vi "Init Splitter.vi"(4 "Maximal size":i16[](array[numeric]), 5 "Label":string, 6 "Minimal size":i16[](array[numeric]), 7 "Vertical? [F, hor.]":bool, 8 "error in (no error)":errorcluster, 9 "Relative size":dbl[](array[numeric]), 10 "Items":refnum<class "IObject.lvclass">[](array[class])) -> (0 "error out":errorcluster, 3 "Splitter out":refnum<class "Splitter.lvclass">)   [LabVIEW 2021, in "Splitter.lvclass"]
doc: "Copyright 2018, Wiebe Walstra, wiebe@carya.nl."
uses:
  Splitter.lvclass
  C:/Projects/Dynamic-Scaling/Dynamic Scaling/IContainer/Divider/Divider.lvclass
  IObject.lvclass
  Divider.lvclass
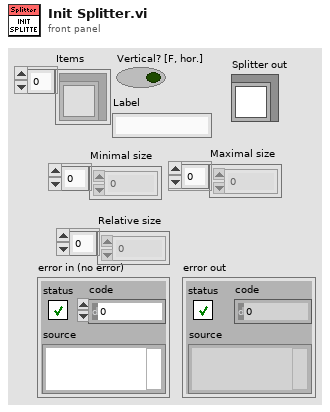
[diagram p1: front panel]
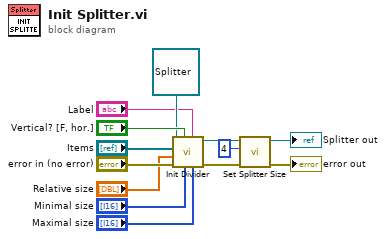
[diagram p0: block diagram]
diagram:
  n1 = call "Init Divider.vi"("Maximal size"="Maximal size", "Label"="Label", "Minimal size"="Minimal size", "Vertical? [F, hor.]"="Vertical? [F, hor.]", "error in (no error)"="error in (no error)", "Relative size"="Relative size", "Items"="Items", "Divider in"=refnum<class "Splitter.lvclass"> refnum ("Splitter in")) -> ("error out"=w6:errorcluster, "Divider out"=w3:refnum<class "Splitter.lvclass">)  [unwired: 2 in]
  n2 = call "Set Splitter Size.vi"("error in (no error)"=w6, "Splitter size [2]"=4 ("Splitter size"), "Divider in"=w3) -> ("error out"=→"error out":errorcluster, "Divider out"=→"Splitter out":refnum<class "Splitter.lvclass">)  [unwired: 7 in]
